vi "Serialize.vi"(7 "DestinationFolder":path, 8 "error in":errorcluster, 9 "OwningElement in":refnum<k20>, 10 "Document in":refnum<k20>, 11 "ProcessRun in":refnum<class "ProcessRun.lvclass">) -> (0 "error out":errorcluster, 1 "OwningElement out":refnum<k20>, 2 "Document out":refnum<k20>, 3 "ProcessRun out":refnum<class "ProcessRun.lvclass">)   [LabVIEW 2021, in "ProligentXMLGenerator.lvlib" / "ProcessRun.lvclass"]
uses:
  ProcessRun.lvclass
  ProcessRun.lvclass/ProcessRun.ctl
  <vilib>/xml/NI_XML.lvlib
  Base/DOMSupport/DOMSupport.lvlib
  OperationRun/OperationRun.lvclass
  OperationCycle/OperationCycle.lvclass
  Model/CustomData/CustomData.lvclass
  Failure/FailureReference/FailureReference.lvclass
  <vilib>/xml/Close Reference(Node).vi
  Base/Guid/Guid.lvclass
  C:/Projects/proligent-xml-generator-labview/src/ProligentXMLGenerator/Base/NonEmptyString/NonEmptyString.lvclass
  C:/Projects/proligent-xml-generator-labview/src/ProligentXMLGenerator/Base/String/String.lvclass
  C:/Projects/proligent-xml-generator-labview/src/ProligentXMLGenerator/Base/Attribute/Attribute.lvclass
  C:/Projects/proligent-xml-generator-labview/src/ProligentXMLGenerator/Base/Guid/Guid.lvclass
  Base/ProcessFullName/ProcessFullName.lvclass
  C:/Projects/proligent-xml-generator-labview/src/ProligentXMLGenerator/Base/ProcessFullName/ProcessFullName.lvclass
  Base/NonEmptyString_64/NonEmptyString_64.lvclass
  C:/Projects/proligent-xml-generator-labview/src/ProligentXMLGenerator/Base/NonEmptyString_64/NonEmptyString_64.lvclass
  Base/NonEmptyString_50/NonEmptyString_50.lvclass
  C:/Projects/proligent-xml-generator-labview/src/ProligentXMLGenerator/Base/NonEmptyString_50/NonEmptyString_50.lvclass
  Base/FullName/FullName.lvclass
  C:/Projects/proligent-xml-generator-labview/src/ProligentXMLGenerator/Base/FullName/FullName.lvclass
  Base/ExecutionStatus/ExecutionStatus.lvclass
  C:/Projects/proligent-xml-generator-labview/src/ProligentXMLGenerator/Base/ExecutionStatus/ExecutionStatus.lvclass
  Base/DateTime/DateTime.lvclass
  C:/Projects/proligent-xml-generator-labview/src/ProligentXMLGenerator/Base/DateTime/DateTime.lvclass
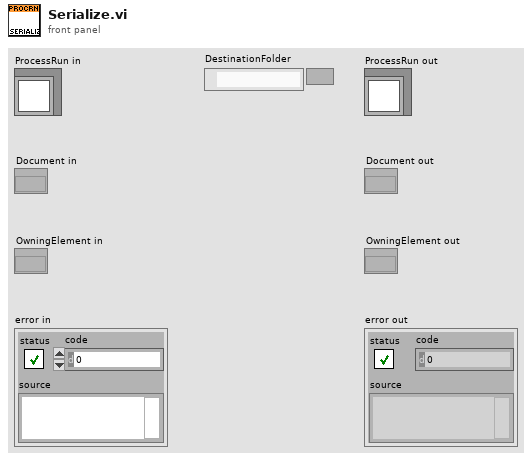
[diagram p1: front panel]
types:
  T1 = typedef "ProligentXMLGenerator.lvlib/ProcessRun.lvclass/Data.ctl" = cluster{"Name":string, "OperationRuns":refnum<class "OperationRun.lvclass">[], "OperationCycles":refnum<class "OperationCycle.lvclass">[], "FailureReferences":refnum<class "FailureReference.lvclass">[], "CustomData":refnum<class "CustomData.lvclass">, "ProcessRunId":refnum<class "Guid.lvclass">, "ProcessFullName":refnum<class "ProcessFullName.lvclass">, "ProcessVersion":refnum<class "NonEmptyString_64.lvclass">, "ProductUnitIdentifier":refnum<class "NonEmptyString_50.lvclass">, "ProductFullName":refnum<class "FullName.lvclass">, "ProcessRunStatus":refnum<class "ExecutionStatus.lvclass">, "ProcessRunStartTime":refnum<class "DateTime.lvclass">, "ProcessRunEndTime":refnum<class "DateTime.lvclass">, "ProcessMode":refnum<class "NonEmptyString_64.lvclass">, "TimeZoneInfoId":string}
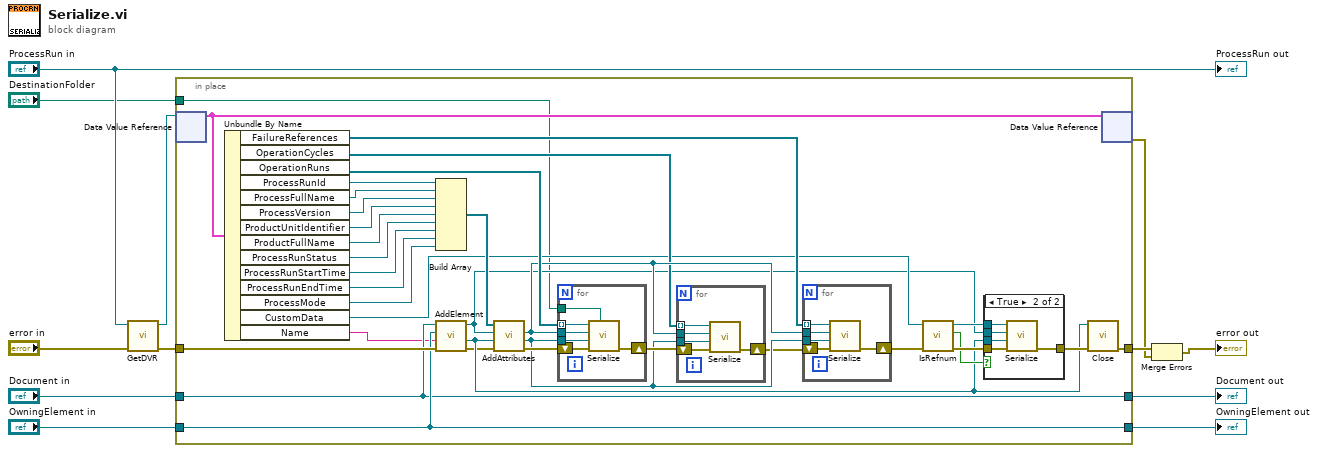
[diagram p0: block diagram]
diagram:
  n1 = call "GetDVR.vi"("error in"="error in", "ProcessRun"="ProcessRun in") -> ("error out"=w4:errorcluster, "DVRReference"=w3:refnum<data-value>)  [unwired: 8 in]
  n2 = in-place "In Place Element Structure" {
    in-place-border: [w46] -> w5
    in-place-border: "Document in" -> [w42]
    in-place-border: w4 -> [w45]
    in-place-border: "OwningElement in" -> [w44]
    in-place-border: [w44] -> w7
    in-place-border: [w42] -> w6
    in-place-border: "DestinationFolder" -> [w13]
    n3 = in-place-dvr #1(w3) -> (w43:T1)  [unwired: 1 out]
    n4 = Unbundle By Name(w43) -> ("FailureReferences"=w20:refnum<class "FailureReference.lvclass">[], "OperationCycles"=w25:refnum<class "OperationCycle.lvclass">[], "OperationRuns"=w41:refnum<class "OperationRun.lvclass">[], "ProcessRunId"=w31:refnum<class "Guid.lvclass">, "ProcessFullName"=w40:refnum<class "ProcessFullName.lvclass">, "ProcessVersion"=w30:refnum<class "NonEmptyString_64.lvclass">, "ProductUnitIdentifier"=w39:refnum<class "NonEmptyString_50.lvclass">, "ProductFullName"=w38:refnum<class "FullName.lvclass">, "ProcessRunStatus"=w37:refnum<class "ExecutionStatus.lvclass">, "ProcessRunStartTime"=w36:refnum<class "DateTime.lvclass">, "ProcessRunEndTime"=w35:refnum<class "DateTime.lvclass">, "ProcessMode"=w34:refnum<class "NonEmptyString_64.lvclass">, "CustomData"=w17:refnum<class "CustomData.lvclass">, "Name"=w21:string)
    n5 = Build Array(w31, w40, w30, w39, w38, w37, w36, w35, w34) -> (w32:refnum<class "Attribute.lvclass">[])
    n6 = call "AddElement.vi"("error in"=w45, "Name"=w21, "OwningElement in"=w44, "Document in"=w42) -> ("error out"=w14:errorcluster, "NewElement"=w16:refnum<k20>, "Document out"=w15:refnum<k20>)  [unwired: 4 in, 1 out]
    n7 = call "AddAttributes.vi"("error in"=w14, "OwningElement in"=w16, "Document in"=w15, "Attributes"=w32) -> ("error out"=w33:errorcluster, "OwningElement out"=w27:refnum<k20>, "Document out"=w28:refnum<k20>)  [unwired: 5 in]
    n8 = for {
      tunnel: w41 -> [w62] mode=indexing
      tunnel: w27 -> [w60]
      tunnel: w28 -> [w61]
      shift-right: [w58] -> w29
      shift-left: w33 -> [w59]
      tunnel: w13 -> [w57]
      n9 = call "Serialize.vi"("DestinationFolder"=w57, "error in"=w59, "OwningElement in"=w60, "Document in"=w61, "OperationRun in"=w62) -> ("error out"=w58:errorcluster)  [unwired: 3 in, 3 out]
    }
    n10 = for {
      tunnel: w25 -> [w52] mode=indexing
      tunnel: w27 -> [w55]
      tunnel: w28 -> [w56]
      shift-right: [w53] -> w26
      shift-left: w29 -> [w54]
      n11 = call "Serialize.vi"("error in"=w54, "OwningElement in"=w55, "Document in"=w56, "OperationCycle in"=w52) -> ("error out"=w53:errorcluster)  [unwired: 4 in, 3 out]
    }
    n12 = for {
      tunnel: w27 -> [w47]
      tunnel: w28 -> [w48]
      shift-right: [w50] -> w19
      shift-left: w26 -> [w51]
      tunnel: w20 -> [w49] mode=indexing
      n13 = call "Serialize.vi"("error in"=w51, "OwningElement in"=w47, "Document in"=w48, "FailureReference in"=w49) -> ("error out"=w50:errorcluster)  [unwired: 4 in, 3 out]
    }
    n14 = call "IsRefnum.vi"("error in"=w19, "CustomDataType in"=w17) -> ("error out"=w24:errorcluster, "IsRefnum"=w22:bool, "CustomDataType out"=w23:refnum<class "CustomData.lvclass">)  [unwired: 7 in]
    n15 = case shown="True" w22 {
      tunnel: w15 -> [_ w65]
      tunnel: w24 -> [w63 w68]
      tunnel: [w63 w67] -> w18
      tunnel: w23 -> [_ w66]
      tunnel: w16 -> [_ w64]
      frame False {
      }
      frame True {
        n16 = call "Serialize.vi"("error in"=w68, "OwningElement in"=w64, "Document in"=w65, "CustomDataType in"=w66) -> ("error out"=w67:errorcluster)  [unwired: 4 in, 3 out]
      }
    }
    n17 = call-poly <vilib>:"Close.vi"("error in (no error)"=w18, "node"=w16) -> ("error out"=w46:errorcluster)  [unwired: 7 in]
    n18 = in-place-dvr #1(w43) -> (w2:errorcluster)  [unwired: 1 out]
  }
  "Document out" <- w6
  "OwningElement out" <- w7
  n19 = Merge Errors(w5, w2) -> (→"error out":errorcluster)
  "ProcessRun out" <- "ProcessRun in"
